vi "ABB configure no load.vi"() -> ()   [LabVIEW 2017]
uses:
  Temp error msg.ctl
  ABB global.vi
panel:
  in  "Temp error":T1="Error: Temperature measurement "
  in  "delete reading":bool
  in  "Temperature Measurement channels":i32(listbox)
  in  "Add reading":bool
  in  "Category":enum16{"None", "Winding", "Ambient"}(ring)
  in  "Temperature Readings":i32(listbox)
  in  "Exit":bool
  in  "No Load Test":T2={"Number Values"=8, "Tolerance (%)"=2.0, "Value (% rated) "=[1.15, 1.0, 0.91, 0.78, 0.66, 0.55, 0.42, 0.3], "Hold time (sec)"=2.0}
  # "Configure No Load Test"
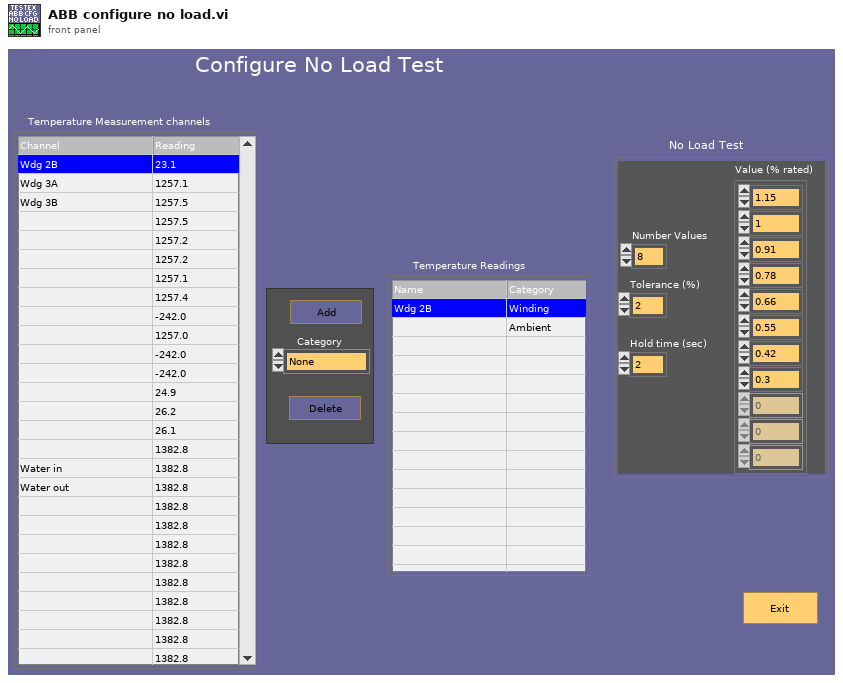
[diagram p1: front panel]
types:
  T1 = typedef "Temp error msg.ctl" = string
  T2 = cluster{"Number Values":i32, "Tolerance (%)":dbl, "Value (% rated) ":dbl[], "Hold time (sec)":dbl}
  T3 = cluster{"temp. alloc":i32[], "category":i32[], "Category names":string[], "Category none names":string[]}
  T4 = cluster{"Number Values":i32, "Tolerance ":dbl, "Value (ratio)":dbl[], "Hold time (sec)":dbl}
  T5 = cluster{"Simulate Norma":bool, "Norma 5000 Address":u8, "WebDaq IP Address":string, "Simulate cDAQ":bool}
  T6 = cluster{"temp. alloc":i32[], "category":i32[], string[], string[]}
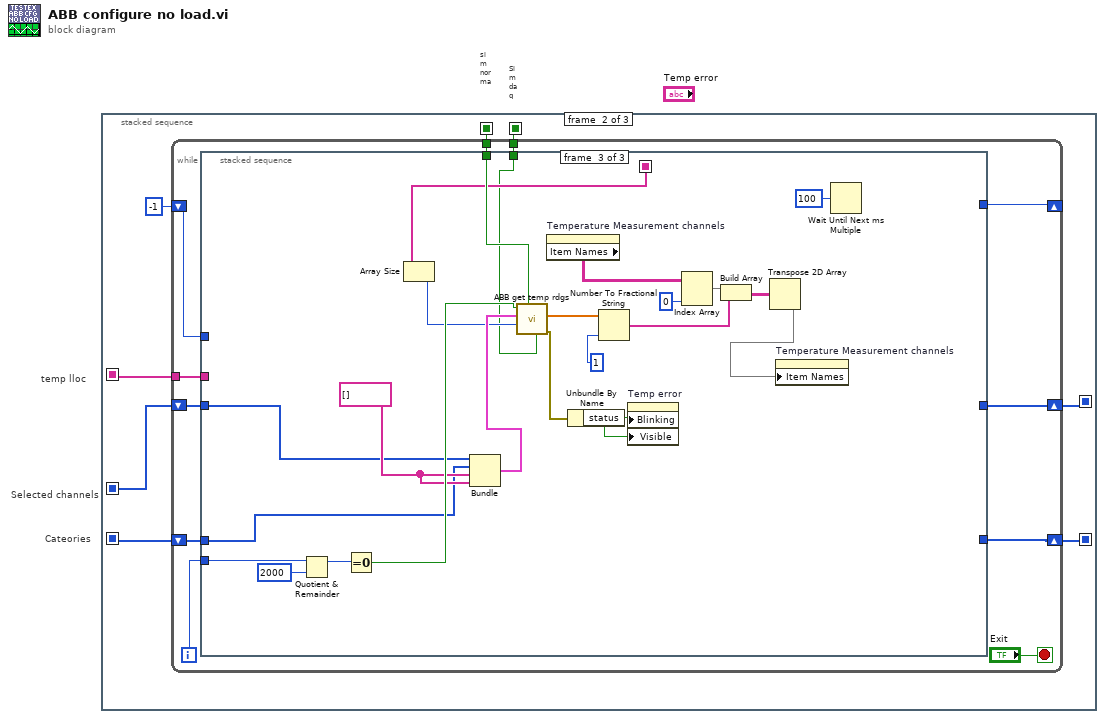
[diagram p0: block diagram]
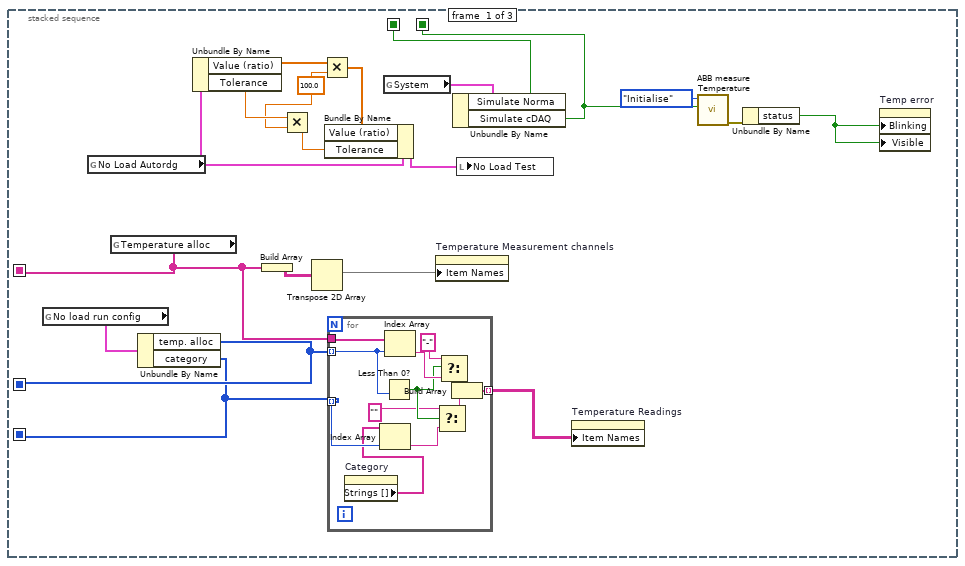
[diagram p2: hidden frame]
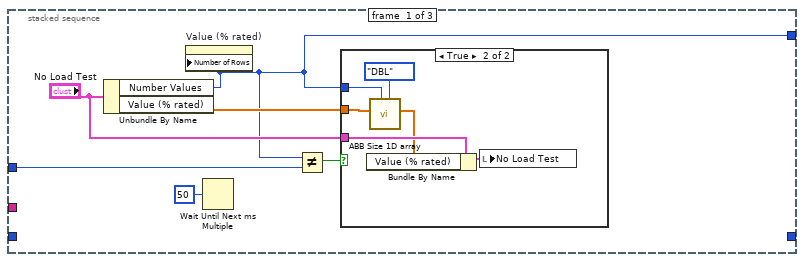
[diagram p3: hidden frame]
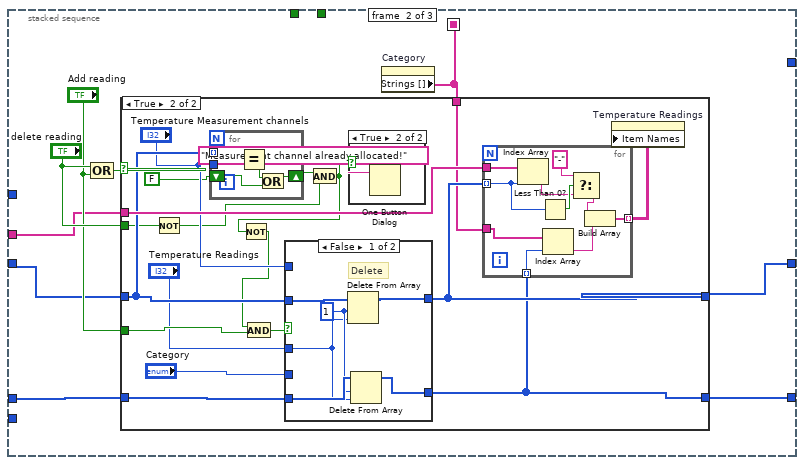
[diagram p5: hidden frame]
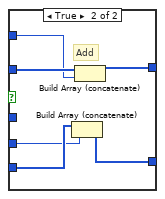
[diagram p8: hidden frame]
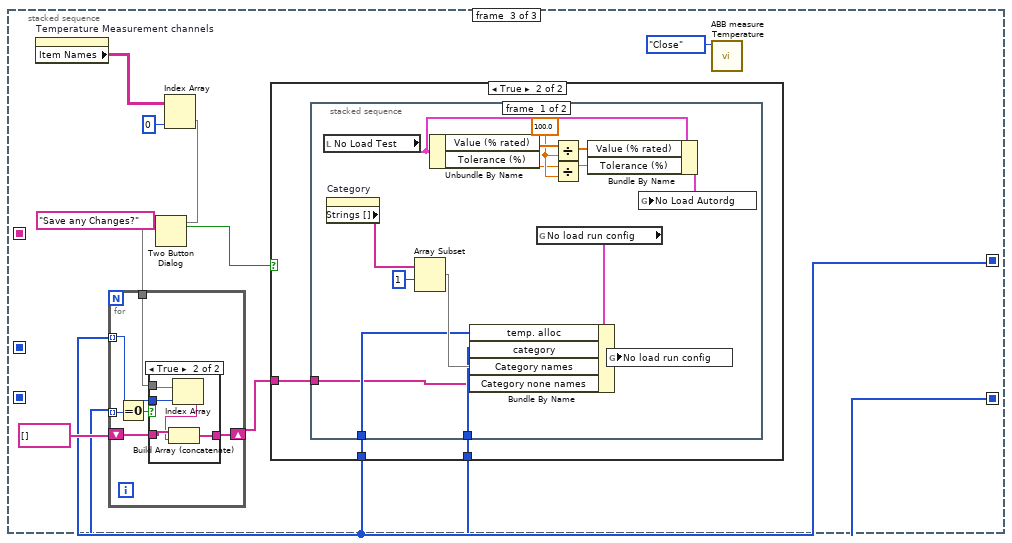
[diagram p9: hidden frame]
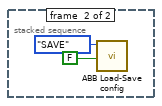
[diagram p12: hidden frame]
diagram:
  # "Sim daq"
  # "sim norma"
  # "temp lloc"
  # "Cateories"
  # "Selected channels"
  n1 = stacked-sequence {
    seq-local: [w12 _ _] -> [_ w39 _]
    seq-local: [w10 _ _] -> [_ w38 _]
    seq-local: [_ w37 _] -> [_ _ w148]
    seq-local: [w7 _ _] -> [_ w36 _]
    seq-local: [w5 _ _] -> [_ w35 _]
    seq-local: [_ w34 _] -> [_ _ w147]
    seq-local: [w4 _ _] -> [_ w33 _]
    frame #0 {
      w15 = 100.0
      n2 = global read "ABB global.vi" "No load run config"() -> (w11:T3)
      n3 = global read "ABB global.vi" "No Load Autordg"() -> (w19:T4)
      n4 = global read "ABB global.vi" "Temperature alloc"() -> (w12:string[])
      n5 = Unbundle By Name(w11) -> ("temp. alloc"=w10:i32[], "category"=w7:i32[])
      n6 = Unbundle By Name(w19) -> ("Value (ratio)"=w20:dbl[], "Tolerance"=w16:dbl)
      n7 = Build Array(w12) -> (w13:string[][])
      n8 = Multiply(x=w16, y=w15) -> (x*y=w14:dbl)
      n9 = Transpose 2D Array(2D array=w13) -> (transposed array=w8:string[][])
      n10 = Multiply(x=w20, y=w15) -> (x*y=w18:dbl[])
      n11 = Bundle By Name(cluster=w19, "Value (ratio)"=w18, "Tolerance"=w14) -> (w17:T4)
      n12 = for {
        tunnel: w12 -> [w32]
        tunnel: w10 -> [w29] mode=indexing
        tunnel: w7 -> [w27] mode=indexing
        tunnel: [w23] -> w9 mode=indexing
        n13 = property on="Category" class="Enum (strict)"() -> ("Strings []"=w21:string[])  [unwired: 2 in, 2 out]
        n14 = Index Array(array=w21, index=w27) -> (element=w26:string)
        n15 = Less Than 0?(x=w29) -> (x < 0?=w28:bool)
        n16 = Index Array(array=w32, index=w29) -> (element=w30:string)
        n17 = Select(t="", s=w28, f=w26) -> (s? t:f=w25:string)
        n18 = Select(t="-", s=w28, f=w30) -> (s? t:f=w24:string)
        n19 = Build Array(w24, w25) -> (w23:string[])
      }
      n20 = global read "ABB global.vi" "System"() -> (w6:T5)
      n21 = property on="Temperature Measurement channels" class="MCListbox (strict)"("Item Names"=w8) -> ()  [unwired: 2 in, 2 out]
      n22 = Unbundle By Name(w6) -> ("Simulate Norma"=w5:bool, "Simulate cDAQ"=w4:bool)
      n23 = local write "No Load Test"(w17) -> ()
      n24 = property on="Temperature Readings" class="MCListbox (strict)"("Item Names"=w9) -> ()  [unwired: 2 in, 2 out]
      n25 = call "ABB measure Temperature.vi"("Simulate"=w4, "Mode"=enum16{"Initialise", "Read", "Close"}."Initialise") -> ("error out"=w2:errorcluster)  [unwired: 7 in, 2 out]
      n26 = Unbundle By Name(w2) -> ("status"=w1:bool)
      n27 = property on="Temp error" class="Str (strict)"("Blinking"=w1, "Visible"=w1) -> ()  [unwired: 2 in, 2 out]
    }
    frame #1 {
      n28 = while {
        shift-right: [w49] -> _
        shift-left: -1 ("Number Values") -> [w50]
        tunnel: w39 -> [w48]
        shift-right: [w46] -> w37
        shift-left: w38 -> [w47]
        shift-right: [w44] -> w34
        shift-left: w36 -> [w45]
        tunnel: w35 -> [w43]
        tunnel: w33 -> [w41]
        i -> [w42]
        stop <- "Exit" stop-if-true
        n29 = stacked-sequence {
          seq-local: [_ w64 _] -> [_ _ w124]
          tunnel: w50 -> [w55 _ _]
          tunnel: [w52 _ _] -> w49
          tunnel: w48 -> [_ w65 _]
          tunnel: w47 -> [_ w69 w131]
          tunnel: [_ w68 _] -> w46
          tunnel: w45 -> [_ w67 w130]
          tunnel: [_ w66 _] -> w44
          tunnel: w43 -> [_ _ w129]
          tunnel: w42 -> [_ _ w126]
          tunnel: w41 -> [_ _ w123]
          frame #0 {
            n30 = Unbundle By Name("No Load Test") -> ("Number Values"=w52:i32, "Value (% rated)"=w53:dbl[])
            n31 = property on="Value (% rated)" class="Arr (strict)"("Number of Rows"=w52) -> ()  [unwired: 2 in, 2 out]
            n32 = Wait Until Next ms Multiple(millisecond multiple=u32 50) -> ()  [unwired: 1 out]
            n33 = Not Equal?(x=w52, y=w55) -> (x != y?=w54:bool)
            n34 = case shown="True" w54 {
              tunnel: "No Load Test" -> [_ w63]
              tunnel: w53 -> [_ w61]
              tunnel: w52 -> [_ w59]
              frame False {
              }
              frame True {
                n35 = call "ABB Size 1D array.vi"("Type"=enum16{"Integer", "DBL", "STRING", "BOOLEAN"}."DBL", "Size"=w59, "DBL Array In"=w61) -> ("DBL Array out"=w58:dbl[])  [unwired: 5 in, 3 out]
                n36 = Bundle By Name(cluster=w63, "Value (% rated)"=w58) -> (w62:T2)
                n37 = local write "No Load Test"(w62) -> ()
              }
            }
          }
          frame #1 {
            n38 = Compound Arithmetic op=OR("delete reading", "Add reading") -> (w72:bool)
            n39 = property on="Category" class="Enum (strict)"() -> ("Strings []"=w64:string[])  [unwired: 2 in, 2 out]
            n40 = case shown="True" w72 {
              tunnel: w69 -> [w74 w88]
              tunnel: [w74 w91] -> w68
              tunnel: w65 -> [_ w92]
              tunnel: "delete reading" -> [_ w81]
              tunnel: w67 -> [w73 w90]
              tunnel: [w73 w89] -> w66
              tunnel: "Add reading" -> [_ w78]
              tunnel: w64 -> [_ w79]
              frame False {
              }
              frame True {
                n41 = Not(x=w81) -> (.not. x?=w80:bool)
                n42 = for {
                  tunnel: w88 -> [w98] mode=indexing
                  tunnel: "Temperature Measurement channels" -> [w97]
                  shift-right: [w94] -> w84
                  shift-left: FALSE -> [w95]
                  n43 = Equal?(x=w98, y=w97) -> (x = y?=w96:bool)
                  n44 = Or(x=w96, y=w95) -> (x .or. y?=w94:bool)
                }
                n45 = And(x=w84, y=w80) -> (x .and. y?=w82:bool)
                n46 = Not(x=w82) -> (.not. x?=w83:bool)
                n47 = And(x=w83, y=w78) -> (x .and. y?=w85:bool)
                n48 = case shown="False" w85 {
                  tunnel: "Category" -> [_ w106]
                  tunnel: "Temperature Measurement channels" -> [_ w108]
                  tunnel: w88 -> [w104 w110]
                  tunnel: [w103 w109] -> w91
                  tunnel: w90 -> [w102 w107]
                  tunnel: [w101 w105] -> w89
                  tunnel: "Temperature Readings" -> [w99 _]
                  frame False {
                    w100 = 1 ("length")
                    # "Delete"
                    n49 = Delete From Array(array=w104, length=w100, index=w99) -> (array with subset deleted=w103:i32[])  [unwired: 1 out]
                    n50 = Delete From Array(array=w102, length=w100, index=w99) -> (array with subset deleted=w101:i32[])  [unwired: 1 out]
                  }
                  frame True {
                    # "Add"
                    n51 = Build Array (concatenate)(w107, w106) -> (w105:i32[])
                    n52 = Build Array (concatenate)(w110, w108) -> (w109:i32[])
                  }
                }
                n53 = case shown="True" w82 {
                  frame False {
                  }
                  frame True {
                    n54 = One Button Dialog(message="Measurement channel already allocated!") -> ()  [unwired: 1 in, 1 out]
                  }
                }
                n55 = for {
                  tunnel: w91 -> [w119] mode=indexing
                  tunnel: w92 -> [w120]
                  tunnel: w79 -> [w114]
                  tunnel: w89 -> [w115] mode=indexing
                  tunnel: [w111] -> w77 mode=indexing
                  n56 = Index Array(array=w120, index=w119) -> (element=w117:string)
                  n57 = Less Than 0?(x=w119) -> (x < 0?=w118:bool)
                  n58 = Index Array(array=w114, index=w115) -> (element=w112:string)
                  n59 = Select(t="-", s=w118, f=w117) -> (s? t:f=w113:string)
                  n60 = Build Array(w113, w112) -> (w111:string[])
                }
                n61 = property on="Temperature Readings" class="MCListbox (strict)"("Item Names"=w77) -> ()  [unwired: 2 in, 2 out]
              }
            }
          }
          frame #2 {
            w133 = string[] []
            n62 = Quotient & Remainder(x=w126, y=2000) -> (x-y*floor(x/y)=w135:i32)  [unwired: 1 out]
            n63 = Equal To 0?(x=w135) -> (x = 0?=w134:bool)
            n64 = Array Size(array=w124) -> (size(s)=w132:i32)
            n65 = Bundle("temp. alloc"=w131, "category"=w130, w133, w133) -> (w143:T6)  [unwired: 1 in]
            n66 = call "ABB get temp rdgs.vi"("Sim daq"=w123, "Simulate norma"=w129, "# categories"=w132, "run config"=w143, "start"=w134) -> ("error out"=w122:errorcluster, "Measured temps"=w142:dbl[])  [unwired: 3 in, 2 out]
            n67 = property on="Temperature Measurement channels" class="MCListbox (strict)"() -> ("Item Names"=w128:string[][])  [unwired: 2 in, 2 out]
            n68 = Unbundle By Name(w122) -> ("status"=w121:bool)
            n69 = Number To Fractional String(number=w142, precision (6)=i16 1) -> (F-format string=w138:string[])  [unwired: 2 in]
            n70 = property on="Temp error" class="Str (strict)"("Blinking"=w121, "Visible"=w121) -> ()  [unwired: 2 in, 2 out]
            n71 = Index Array(array=w128, index (col)=0 ("disabled index (col)")) -> (element=w139:string[])  [unwired: 1 in]
            n72 = Build Array(w139, w138) -> (w137:string[][])
            n73 = Transpose 2D Array(2D array=w137) -> (transposed array=w127:string[][])
            n74 = property on="Temperature Measurement channels" class="MCListbox (strict)"("Item Names"=w127) -> ()  [unwired: 2 in, 2 out]
            n75 = Wait Until Next ms Multiple(millisecond multiple=u32 100) -> ()  [unwired: 1 out]
          }
        }
      }
    }
    frame #2 {
      n76 = property on="Temperature Measurement channels" class="MCListbox (strict)"() -> ("Item Names"=w146:string[][])  [unwired: 2 in, 2 out]
      n77 = Two Button Dialog(message="Save any Changes?") -> (T button?=w153:bool)  [unwired: 2 in]
      n78 = Index Array(array=w146, index (col)=0 ("disabled index (col)")) -> (element=w150:string[])  [unwired: 1 in]
      n79 = for {
        tunnel: w148 -> [w156] mode=indexing
        tunnel: w147 -> [w158] mode=indexing
        tunnel: w150 -> [w157]
        shift-right: [w154] -> w145
        shift-left: string[] [] -> [w155]
        n80 = Equal To 0?(x=w158) -> (x = 0?=w159:bool)
        n81 = case shown="True" w159 {
          tunnel: w157 -> [_ w165]
          tunnel: w156 -> [_ w164]
          tunnel: [w160 w163] -> w154
          tunnel: w155 -> [w160 w162]
          frame False {
          }
          frame True {
            n82 = Index Array(array=w165, index=w164) -> (element=w161:string)
            n83 = Build Array (concatenate)(w162, w161) -> (w163:string[])
          }
        }
      }
      n84 = case shown="True" w153 {
        tunnel: w148 -> [_ w168]
        tunnel: w147 -> [_ w167]
        tunnel: w145 -> [_ w166]
        frame False {
        }
        frame True {
          n85 = stacked-sequence {
            tunnel: w168 -> [w172 _]
            tunnel: w167 -> [w171 _]
            tunnel: w166 -> [w170 _]
            frame #0 {
              w178 = 100.0 ("Numeric")
              n86 = local read "No Load Test"() -> (w181:T2)
              n87 = property on="Category" class="Enum (strict)"() -> ("Strings []"=w169:string[])  [unwired: 2 in, 2 out]
              n88 = Array Subset(array=w169, index=1) -> (w174:string[])  [unwired: 1 in]
              n89 = Unbundle By Name(w181) -> ("Value (% rated)"=w183:dbl[], "Tolerance (%)"=w177:dbl)
              n90 = global read "ABB global.vi" "No load run config"() -> (w176:T3)
              n91 = Bundle By Name(cluster=w176, "temp. alloc"=w172, "category"=w171, "Category names"=w174, "Category none names"=w170) -> (w175:T3)
              n92 = Divide(x=w183, y=w178) -> (x/y=w182:dbl[])
              n93 = Divide(x=w177, y=w178) -> (x/y=w179:dbl)
              n94 = Bundle By Name(cluster=w181, "Value (% rated)"=w182, "Tolerance (%)"=w179) -> (w180:T2)
              n95 = global write "ABB global.vi" "No load run config"(w175) -> ()
              n96 = global write "ABB global.vi" "No Load Autordg"(w180) -> ()
            }
            frame #1 {
              n97 = call "ABB Load-Save config.vi"("confirm save"=FALSE, "Mode"=enum16{"LOAD", "SAVE"}."SAVE") -> ()  [unwired: 10 in]
            }
          }
        }
      }
      n98 = call "ABB measure Temperature.vi"("Mode"=enum16{"Initialise", "Read", "Close"}."Close") -> ()  [unwired: 8 in, 3 out]
    }
  }
